vi "LIDAR Panning.vi"   [LabVIEW 2014]
types:
  T1 = typedef "WPI_ServoDeviceRef.ctl" = cluster{"DeviceStatus":errorcluster, "Controller":T2, "PWM Channel":T3, "DeadBand":T4}
  T2 = typedef "FPGA_TypedefDigitalModule.ctl" = enum16{"Controller 1"}
  T3 = typedef "FPGA_DIOPWMChannel.ctl" = enum8{"PWM 0", "PWM 1", "PWM 2", "PWM 3", "PWM 4", "PWM 5", "PWM 6", "PWM 7", "PWM 8", "PWM 9", "PWM MXP 0", "PWM MXP 1", "PWM MXP 2", "PWM MXP 3", "PWM MXP 4", "PWM MXP 5", "PWM MXP 6", "PWM MXP 7", "PWM MXP 8", "PWM MXP 9", "Invalid"}
  T4 = typedef "WPI_PWMDeadband.ctl" = cluster{"Name":string, "maxPositivePwm":i32, "minPositivePwm":i32, "centerPwm":i32, "maxNegativePwm":i32, "minNegativePwm":i32, "angularRange":u16}
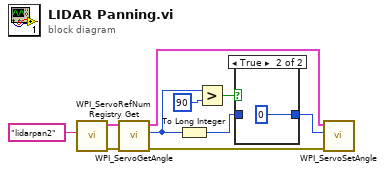
[diagram p0: block diagram]
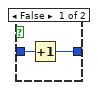
[diagram p2: hidden frame]
diagram:
  n1 = call <vilib>:"WPI_ServoRefNum Registry Get.vi"("refnum name"="lidarpan2") -> ("error out"=w9:errorcluster, "ServoDeviceRef"=w8:T1)  [unwired: 9 in]
  n2 = call <vilib>:"WPI_ServoGetAngle.vi"("ServoDeviceRef"=w8, "error in (no error)"=w9) -> ("ServoDeviceRef"=w5:T1, "Angle"=w2:u16, "error out"=w6:errorcluster)  [unwired: 6 in]
  n3 = To Long Integer(number=w2) -> (32bit integer=w3:i32)
  n4 = Greater?(x=w2, y=u16 90 ("x")) -> (0:w7:bool)
  n5 = case shown="True" w7 {
    tunnel: w3 -> [w12 _]
    tunnel: [w11 0] -> w4
    frame False {
      n6 = Increment(x=w12) -> (x+1=w11:i32)
    }
    frame True {
    }
  }
  n7 = call <vilib>:"WPI_ServoSetAngle.vi"("error in (no error)"=w6, "Angle"=w4, "ServoDeviceRef"=w5) -> ()  [unwired: 7 in, 2 out]
